vi "Stream Delay.vi"(7 "Delay Time (0)":u32, 8 "error in (no error)":errorcluster, 9 "Device Number":string, 10 "Stream Number (1)":u8=1, 11 "VISA resource name":refnum<visa-resource-name>) -> (0 "error out":errorcluster, 3 "VISA resource name out":refnum<visa-resource-name>)   [LabVIEW 2015, in "Zaber A Series.lvlib"]
doc: "Inserts a delay into a stream. Device motion will stop for the specified number of milliseconds.\n\nThis VI does not check in advance for error conditions such as streams not being supported.\n\nThis VI requires that the Initialize VI has been called with the same serial port."
uses:
  Zaber A Series.lvlib
  Private/All Commands.ctl
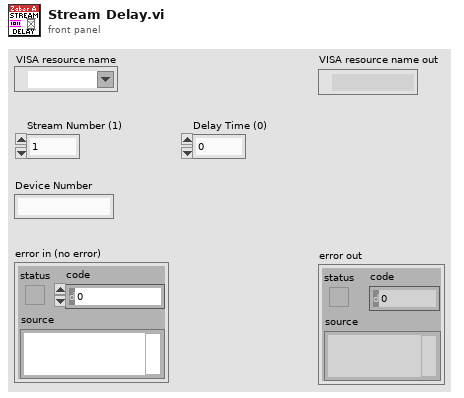
[diagram p1: front panel]
types:
  T1 = typedef "Zaber A Series.lvlib/All Commands.ctl" = string
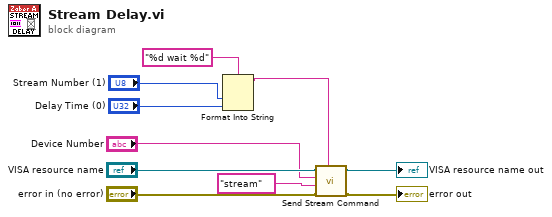
[diagram p0: block diagram]
diagram:
  n1 = Format Into String(format string="%d wait %d", "Stream Number (1)", "Delay Time (0)") -> (resulting string=w2:string)  [unwired: 2 in, 1 out]
  n2 = call "Send Stream Command.vi"("Data"=w2, "error in (no error)"="error in (no error)", "Command"=T1 "stream" ("Complete Command List"), "Device Number"="Device Number", "VISA resource name"="VISA resource name") -> ("error out"=→"error out":errorcluster, "VISA resource name out"=→"VISA resource name out":refnum<visa-resource-name>)  [unwired: 5 in]
